vi "F.vi"(9 "String":string, 10 "format string":string, 11 "result string in":string) -> (3 "result string out":string)   [LabVIEW 2017]
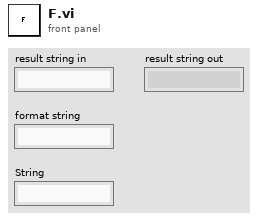
[diagram p1: front panel]
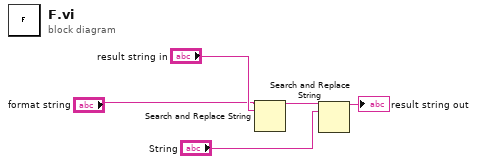
[diagram p0: block diagram]
diagram:
  n1 = Search and Replace String(input string="format string", search string="result string in") -> (result string=w3:string)  [unwired: 6 in, 3 out]
  n2 = Search and Replace String(input string=w3, search string="String") -> (result string=→"result string out":string)  [unwired: 6 in, 3 out]
